vi "Translator.File.Write.vi"(8 "error in":errorcluster, 10 "Language in use":string, 11 "Translation folder":path=path "D:/PL_0125_Sapphire_Automation/settings") -> (0 "error out":errorcluster)   [LabVIEW 2019, in "Tools.lvlib"]
uses:
  Tools.lvlib
  Translator.Enums.ctl
  <vilib>/Utility/config.llb/Read Key (String).vi
  <vilib>/Utility/config.llb/Write Key (String).vi
  <vilib>/Utility/config.llb/NI_LVConfig.lvlib
panel:
  in  "Enums":T1
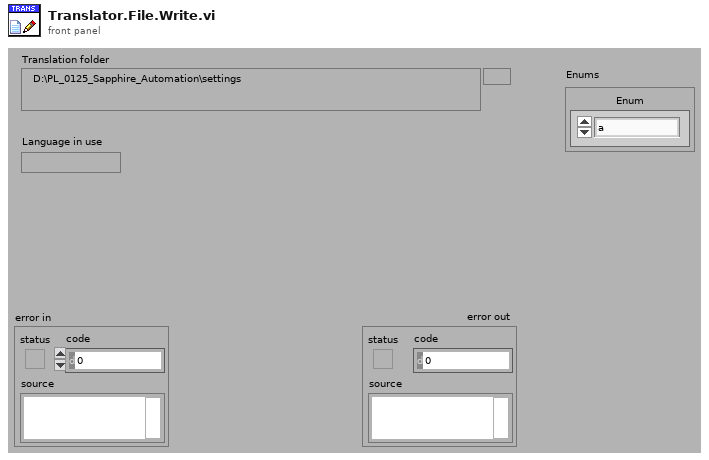
[diagram p1: front panel]
types:
  T1 = typedef "Tools.lvlib/Translator.Enums.ctl" = cluster{"Enum":enum16{"a", "b", "c"}}
  T2 = typedef "NI_LVConfig.lvlib/Config Data RefNum.ctl" = refnum<k1>
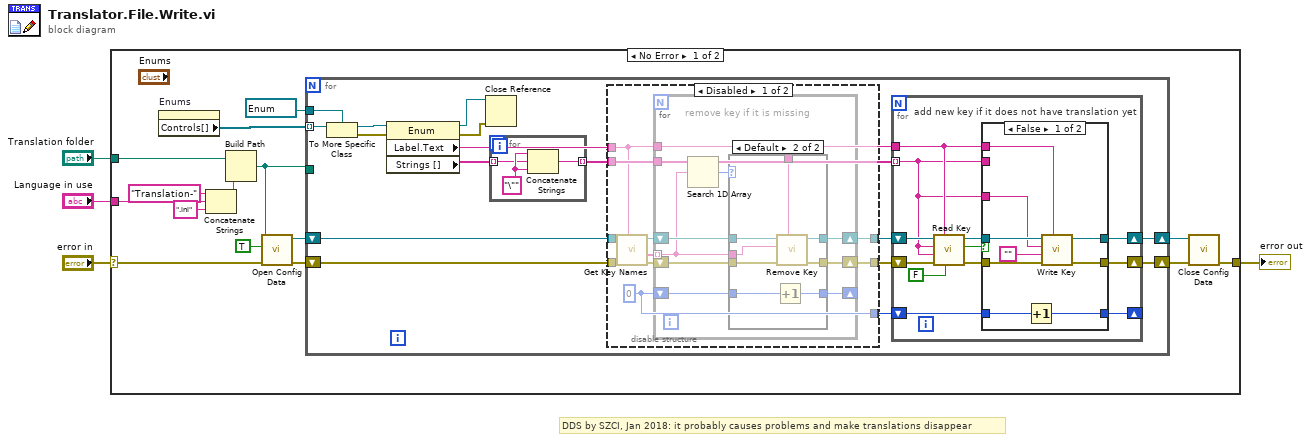
[diagram p0: block diagram]
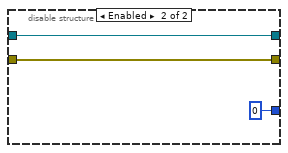
[diagram p3: hidden frame]
diagram:
  # "DDS by SZCI, Jan 2018: it probably causes problems and make translations disappear"
  n1 = case shown="No Error" "error in" {
    selector: "error in" -> [w12 w97]
    tunnel: "Translation folder" -> [w19 _]
    tunnel: [w6 w97] -> w3
    tunnel: "Language in use" -> [w18 _]
    frame No Error {
      n2 = property on="Enums" class="Clust (strict)"() -> ("Controls[]"=w14:refnum<vi>[])  [unwired: 2 in, 2 out]
      n3 = Concatenate Strings("Translation-" ("string"), w18, ".ini" ("string")) -> (w17:string)
      n4 = Build Path(base path=w19, name or relative path=w17) -> (appended path=w11:path)
      n5 = call <vilib>:"Open Config Data.vi"("error in (no error)"=w12, "create file if necessary (T)"=TRUE, "configuration file path"=w11) -> ("error out"=w10:errorcluster, "refnum"=w9:T2)  [unwired: 6 in, 1 out]
      n6 = for {
        shift-right: [w22] -> w7
        shift-left: w10 -> [w31]
        tunnel: w14 -> [w30] mode=indexing
        tunnel: w11 -> [_]
        tunnel: refnum<vi> refnum ("reference out") -> [w27]
        shift-right: [w23] -> w8
        shift-left: w9 -> [w24]
        n7 = To More Specific Class(target class=w27, reference=w30) -> (specific class reference=w29:refnum<vi>, error out=w28:errorcluster)  [unwired: 1 in]
        n8 = property class="Enum"(reference=w29, error in=w28) -> (reference out=w20:refnum<vi>, error out=w21:errorcluster, "Label.Text"=w25:string, "Strings []"=w26:string[])
        n9 = Close Reference(reference=w20, error in (no error)=w21) -> ()  [unwired: 1 out]
        n10 = for {
          tunnel: w26 -> [w71] mode=indexing
          tunnel: [w70] -> w32 mode=indexing
          w72 = "\""
          n11 = Concatenate Strings(w72, w71, w72) -> (w70:string)
        }
        n12 = disable-structure shown="Disabled" {
          disable-tunnel: [w44 w68] -> w35
          disable-tunnel: [w43 w69] -> w34
          disable-tunnel: [w40 0] -> w33
          disable-tunnel: w32 -> [w39 _]
          disable-tunnel: w31 -> [w38 w68]
          disable-tunnel: w25 -> [w37 _]
          disable-tunnel: w24 -> [w36 w69]
          frame Disabled {
            w40 = 0
            n13 = call <vilib>:"Get Key Names.vi"("section"=w37, "error in (no error)"=w38, "refnum"=w36) -> ("error out"=w45:errorcluster, "key names"=w41:string[], "refnum out"=w42:T2)  [unwired: 5 in, 1 out]
            n14 = for {
              shift-right: [w52] -> w44
              shift-left: w45 -> [w55]
              shift-right: [w54] -> w43
              shift-left: w42 -> [w53]
              tunnel: w41 -> [w50] mode=indexing
              tunnel: w39 -> [w51]
              tunnel: w37 -> [w48]
              shift-right: [w46] -> _
              shift-left: w40 -> [w47]
              # "remove key if it is missing"
              n15 = Search 1D Array(1D array=w51, element=w50) -> (index of element=w49:i32)  [unwired: 1 in]
              n16 = case shown="Default" w49 {
                tunnel: w55 -> [w58 w66]
                tunnel: [w57 w65] -> w54
                tunnel: w53 -> [w57 w64]
                tunnel: w50 -> [_ w63]
                tunnel: [w58 w62] -> w52
                tunnel: w48 -> [_ w61]
                tunnel: w47 -> [w56 w60]
                tunnel: [w56 w59] -> w46
                frame 0.. {
                }
                frame Default {
                  n17 = Increment(x=w60) -> (x+1=w59:i32)
                  n18 = call <vilib>:"Remove Key.vi"("section"=w61, "error in (no error)"=w66, "key"=w63, "refnum"=w64) -> ("error out"=w62:errorcluster, "refnum out"=w65:T2)  [unwired: 5 in, 1 out]
                }
              }
            }
          }
          frame Enabled {
          }
        }
        n19 = for {
          tunnel: w25 -> [w80]
          tunnel: w32 -> [w73] mode=indexing
          shift-right: [w84] -> w22
          shift-left: w35 -> [w81]
          shift-right: [w83] -> w23
          shift-left: w34 -> [w82]
          shift-right: [w75] -> _
          shift-left: w33 -> [w76]
          # "add new key if it does not have translation yet"
          n20 = call-poly <vilib>:"Read Key.vi"("read raw string? (F)"=FALSE, "section"=w80, "error in (no error)"=w81, "default value"=w73, "key"=w73, "refnum"=w82) -> ("error out"=w77:errorcluster, "found?"=w79:bool, "refnum out"=w78:T2)  [unwired: 2 in, 1 out]
          n21 = case shown="False" w79 {
            tunnel: [w93 w95] -> w84
            tunnel: [w92 w96] -> w83
            tunnel: w78 -> [w91 w96]
            tunnel: w77 -> [w90 w95]
            tunnel: w80 -> [w89 _]
            tunnel: w73 -> [_ _]
            tunnel: [w86 w94] -> w75
            tunnel: w76 -> [w87 w94]
            tunnel: w73 -> [w85 _]
            frame False {
              n22 = Increment(x=w87) -> (x+1=w86:i32)
              n23 = call-poly <vilib>:"Write Key.vi"("section"=w89, "error in (no error)"=w90, "value"="", "key"=w85, "refnum"=w91) -> ("error out"=w93:errorcluster, "refnum out"=w92:T2)  [unwired: 4 in, 1 out]
            }
            frame True {
            }
          }
        }
      }
      n24 = call <vilib>:"Close Config Data.vi"("error in (no error)"=w7, "refnum"=w8) -> ("error out"=w6:errorcluster)  [unwired: 8 in, 1 out]
    }
    frame Error {
    }
  }
  "error out" <- w3
